vi "RampVoltagewithDDSv11.vi"() -> ()   [LabVIEW 2016]
uses:
  <vilib>/DAQmx/write.llb/DAQmx Write (Digital 1D Wfm NChan NSamp).vi
  <vilib>/DAQmx/write.llb/DAQmx Write (Analog 2D DBL NChan NSamp).vi
  <vilib>/DAQmx/create/channels.llb/DAQmx Create Channel (AO-Voltage-Basic).vi
  <vilib>/DAQmx/create/channels.llb/DAQmx Create Channel (DO-Digital Output).vi
  <vilib>/DAQmx/configure/timing.llb/DAQmx Timing (Sample Clock).vi
  <vilib>/DAQmx/configure/trigger.llb/DAQmx Start Trigger (Digital Edge).vi
  <vilib>/DAQmx/miscellaneous.llb/DAQmx Fill In Error Info.vi
  <vilib>/Waveform/DWDTOps.llb/DWDT Boolean Array to Digital.vi
  <vilib>/Waveform/DWDTOps.llb/DWDT Uncompress Digital.vi
  <vilib>/Waveform/DTblOps.llb/DTbl Digital to Analog.vi
  <resource>/objmgr/daqmx.rc
panel:
  in  "High/Low":bool
  in  "Reset P0.1":bool
  in  "Constant PO.0?":bool
  in  "DDS Trigger delay (ms)":dbl=0.5 step=0.01
  in  "DDS Trigger (Port 0 Line 1)":tag="Dev2/port0/line1"
  out "Digital Output":cluster{i32, dbl, dbl[][]}(graph)={0, 1e-05, [[0.0, 0.0, 0.0, 0.0, 0.0, 0.0, 0.0, 0.0, 0.0, 0.0, 0.0, 0.0, 0.0, 0.0, 0.0, 0.0, 0.0, 0.0, 0.0, 0.0, 0.0, 0.0, 0.0, 0.0, 0.0, 0.0, 0.0, 0.0, 0.0, 0.0, 0.0, 0.0, 0.0, 0.0, 0.0, 0.0, 0.0, 0.0, 0.0, 0.0, 0.0, 0.0, 0.0, 0.0, 0.0, 0.0, 0.0, 0.0, 0.0, 0.0, 0.0, 0.0, 0.0, 0.0, 0.0, 0.0, 0.0, 0.0, 0.0, 0.0, 0.0, 0.0, 0.0, 0.0, 0.0, 0.0, 0.0, 0.0, 0.0, 0.0, 0.0, 0.0, 0.0, 0.0, 0.0, 0.0, 0.0, 0.0, 0.0, 0.0, 0.0, 0.0, 0.0, 0.0, 0.0, 0.0, 0.0, 0.0, 0.0, 0.0, 0.0, 0.0, 0.0, 0.0, 0.0, 0.0, 0.0, 0.0, 0.0, 0.0, 5.0, 5.0, 5.0, 5.0, 5.0, 5.0, 5.0, 5.0, 5.0, 5.0, 5.0, 5.0, 5.0, 5.0, 5.0, 5.0, 5.0, 5.0, 5.0, 5.0, 5.0, 5.0, 5.0, 5.0, 5.0, 5.0, 5.0, 5.0, 5.0, 5.0, 5.0, 5.0, 5.0, 5.0, 5.0, 5.0, 5.0, 5.0, 5.0, 5.0, 5.0, 5.0, 5.0, 5.0, 5.0, 5.0, 5.0, 5.0, 5.0, 5.0, 5.0, 5.0, 5.0, 5.0, 5.0, 5.0, 5.0, 5.0, 5.0, 5.0, 5.0, 5.0, 5.0, 5.0, 5.0, 5.0, 5.0, 5.0, 5.0, 5.0, 5.0, 5.0, 5.0, 5.0, 5.0, 5.0, 5.0, 5.0, 5.0, 5.0, 5.0, 5.0, 5.0, 5.0, 5.0, 5.0, 5.0, 5.0, 5.0, 5.0, 5.0, 5.0, 5.0, 5.0, 5.0, 5.0, 5.0, 5.0, 5.0, 5.0, 5.0, 5.0, 5.0, 5.0, 5.0, 5.0, 5.0, 5.0, 5.0, 5.0, 5.0, 5.0, 5.0, 5.0, 5.0, 5.0, 5.0, 5.0, 5.0, 5.0, 5.0, 5.0, 5.0, 5.0, 5.0, 5.0, 5.0, 5.0, 5.0, 5.0, 5.0, 5.0, 5.0, 5.0, 5.0, 5.0, 5.0, 5.0, 5.0, 5.0, 5.0, 5.0, 5.0, 5.0, 5.0, 5.0, 5.0, 5.0, 5.0, 5.0, 5.0, 5.0, 5.0, 5.0, 5.0, 5.0, 5.0, 5.0, 5.0, 5.0, 5.0, 5.0, 5.0, 5.0, 5.0, 5.0, 5.0, 5.0, 5.0, 5.0, 5.0, 5.0, 5.0, 5.0, 5.0, 5.0, 5.0, 5.0, 5.0, 5.0, 5.0, 5.0, 5.0, 5.0, 5.0, 5.0, 5.0, 5.0, 5.0, 5.0, 5.0, 5.0, 5.0, 5.0, 5.0, 5.0, 5.0, 5.0, 5.0, 5.0, 0.0, 0.0, 0.0, 0.0, 0.0, 0.0, 0.0, 0.0, 0.0, 0.0, 0.0, 0.0, 0.0, 0.0, 0.0, 0.0, 0.0, 0.0, 0.0, 0.0, 0.0, 0.0, 0.0, 0.0, 0.0, 0.0, 0.0, 0.0, 0.0, 0.0, 0.0, 0.0, 0.0, 0.0, 0.0, 0.0, 0.0, 0.0, 0.0, 0.0, 0.0, 0.0, 0.0, 0.0, 0.0, 0.0, 0.0, 0.0, 0.0, 0.0, 0.0, 0.0, 0.0, 0.0, 0.0, 0.0, 0.0, 0.0, 0.0, 0.0, 0.0, 0.0, 0.0, 0.0, 0.0, 0.0, 0.0, 0.0, 0.0, 0.0, 0.0, 0.0, 0.0, 0.0, 0.0, 0.0, 0.0, 0.0, 0.0, 0.0, 0.0, 0.0, 0.0, 0.0, 0.0, 0.0, 0.0, 0.0, 0.0, 0.0, 0.0, 0.0, 0.0, 0.0, 0.0, 0.0, 0.0, 0.0, 0.0, 0.0, 0.0, 0.0, 0.0, 0.0, 0.0, 0.0, 0.0, 0.0, 0.0, 0.0, 0.0, 0.0, 0.0, 0.0, 0.0, 0.0, 0.0, 0.0, 0.0, 0.0, 0.0, 0.0, 0.0, 0.0, 0.0, 0.0, 0.0, 0.0, 0.0, 0.0, 0.0, 0.0, 0.0, 0.0, 0.0, 0.0, 0.0, 0.0, 0.0, 0.0, 0.0, 0.0, 0.0, 0.0, 0.0, 0.0, 0.0, 0.0, 0.0, 0.0, 0.0, 0.0, 0.0, 0.0, 0.0, 0.0, 0.0, 0.0, 0.0, 0.0, 0.0, 0.0, 0.0, 0.0, 0.0, 0.0, 0.0, 0.0, 0.0, 0.0, 0.0, 0.0, 0.0, 0.0, 0.0, 0.0, 0.0, 0.0, 0.0, 0.0, 0.0, 0.0, 0.0, 0.0, 0.0, 0.0, 0.0, 0.0, 0.0, 0.0, 0.0, 0.0, 0.0, 0.0, 0.0, 0.0, 0.0, 0.0, 0.0, 0.0, 5.0, 5.0, 5.0, 5.0, 5.0, 5.0, 5.0, 5.0, 5.0, 5.0, 5.0, 5.0, 5.0, 5.0, 5.0, 5.0, 5.0, 5.0, 5.0, 5.0, 5.0, 5.0, 5.0, 5.0, 5.0, 5.0, 5.0, 5.0, 5.0, 5.0, 5.0, 5.0, 5.0, 5.0, 5.0, 5.0, 5.0, 5.0, 5.0, 5.0, 5.0, 5.0, 5.0, 5.0, 5.0, 5.0, 5.0, 5.0, 5.0, 5.0, 5.0, 5.0, 5.0, 5.0, 5.0, 5.0, 5.0, 5.0, 5.0, 5.0, 5.0, 5.0, 5.0, 5.0, 5.0, 5.0, 5.0, 5.0, 5.0, 5.0, 5.0, 5.0, 5.0, 5.0, 5.0, 5.0, 5.0, 5.0, 5.0, 5.0, 5.0, 5.0, 5.0, 5.0, 5.0, 5.0, 5.0, 5.0, 5.0, 5.0, 5.0, 5.0, 5.0, 5.0, 5.0, 5.0, 5.0, 5.0, 5.0, 5.0, 5.0, 5.0, 5.0, 5.0, 5.0, 5.0, 5.0, 5.0, 5.0, 5.0, 5.0, 5.0, 5.0, 5.0, 5.0, 5.0, 5.0, 5.0, 5.0, 5.0, 5.0, 5.0, 5.0, 5.0, 5.0, 5.0, 5.0, 5.0, 5.0, 5.0, 5.0, 5.0, 5.0, 5.0, 5.0, 5.0, 5.0, 5.0, 5.0, 5.0, 5.0, 5.0, 5.0, 5.0, 5.0, 5.0, 5.0, 5.0, 5.0, 5.0, 5.0, 5.0, 5.0, 5.0, 5.0, 5.0, 5.0, 5.0, 5.0, 5.0, 5.0, 5.0, 5.0, 5.0, 5.0, 5.0, 5.0, 5.0, 5.0, 5.0, 5.0, 5.0, 5.0, 5.0, 5.0, 5.0, 5.0, 5.0, 5.0, 5.0, 5.0, 5.0, 5.0, 5.0, 5.0, 5.0, 5.0, 5.0, 5.0, 5.0, 5.0, 5.0, 5.0, 5.0, 5.0, 5.0, 5.0, 5.0, 5.0, 5.0, 0.0, 0.0, 0.0, 0.0, 0.0, 0.0, 0.0, 0.0, 0.0, 0.0, 0.0, 0.0, 0.0, 0.0, 0.0, 0.0, 0.0, 0.0, 0.0, 0.0, 0.0, 0.0, 0.0, 0.0, 0.0, 0.0, 0.0, 0.0, 0.0, 0.0, 0.0, 0.0, 0.0, 0.0, 0.0, 0.0, 0.0, 0.0, 0.0, 0.0, 0.0, 0.0, 0.0, 0.0, 0.0, 0.0, 0.0, 0.0, 0.0, 0.0, 0.0, 0.0, 0.0, 0.0, 0.0, 0.0, 0.0, 0.0, 0.0, 0.0, 0.0, 0.0, 0.0, 0.0, 0.0, 0.0, 0.0, 0.0, 0.0, 0.0, 0.0, 0.0, 0.0, 0.0, 0.0, 0.0, 0.0, 0.0, 0.0, 0.0, 0.0, 0.0, 0.0, 0.0, 0.0, 0.0, 0.0, 0.0, 0.0, 0.0, 0.0, 0.0, 0.0, 0.0, 0.0, 0.0, 0.0, 0.0, 0.0, 0.0, 5.0], [5.0, 5.0, 5.0, 5.0, 5.0, 5.0, 5.0, 5.0, 5.0, 5.0, 5.0, 5.0, 5.0, 5.0, 5.0, 5.0, 5.0, 5.0, 5.0, 5.0, 5.0, 5.0, 5.0, 5.0, 5.0, 5.0, 5.0, 5.0, 5.0, 5.0, 5.0, 5.0, 5.0, 5.0, 5.0, 5.0, 5.0, 5.0, 5.0, 5.0, 5.0, 5.0, 5.0, 5.0, 5.0, 5.0, 5.0, 5.0, 5.0, 5.0, 5.0, 5.0, 5.0, 5.0, 5.0, 5.0, 5.0, 5.0, 5.0, 5.0, 5.0, 5.0, 5.0, 5.0, 5.0, 5.0, 5.0, 5.0, 5.0, 5.0, 5.0, 5.0, 5.0, 5.0, 5.0, 5.0, 5.0, 5.0, 5.0, 5.0, 5.0, 5.0, 5.0, 5.0, 5.0, 5.0, 5.0, 5.0, 5.0, 5.0, 5.0, 5.0, 5.0, 5.0, 5.0, 5.0, 5.0, 5.0, 5.0, 5.0, 5.0, 5.0, 5.0, 5.0, 5.0, 5.0, 5.0, 5.0, 5.0, 5.0, 5.0, 5.0, 5.0, 5.0, 5.0, 5.0, 5.0, 5.0, 5.0, 5.0, 5.0, 5.0, 5.0, 5.0, 5.0, 5.0, 5.0, 5.0, 5.0, 5.0, 5.0, 5.0, 5.0, 5.0, 5.0, 5.0, 5.0, 5.0, 5.0, 5.0, 5.0, 5.0, 5.0, 5.0, 5.0, 5.0, 5.0, 5.0, 5.0, 5.0, 0.0, 0.0, 0.0, 0.0, 0.0, 0.0, 0.0, 0.0, 0.0, 0.0, 0.0, 0.0, 0.0, 0.0, 0.0, 0.0, 0.0, 0.0, 0.0, 0.0, 0.0, 0.0, 0.0, 0.0, 0.0, 0.0, 0.0, 0.0, 0.0, 0.0, 0.0, 0.0, 0.0, 0.0, 0.0, 0.0, 0.0, 0.0, 0.0, 0.0, 0.0, 0.0, 0.0, 0.0, 0.0, 0.0, 0.0, 0.0, 0.0, 0.0, 0.0, 0.0, 0.0, 0.0, 0.0, 0.0, 0.0, 0.0, 0.0, 0.0, 0.0, 0.0, 0.0, 0.0, 0.0, 0.0, 0.0, 0.0, 0.0, 0.0, 0.0, 0.0, 0.0, 0.0, 0.0, 0.0, 0.0, 0.0, 0.0, 0.0, 0.0, 0.0, 0.0, 0.0, 0.0, 0.0, 0.0, 0.0, 0.0, 0.0, 0.0, 0.0, 0.0, 0.0, 0.0, 0.0, 0.0, 0.0, 0.0, 0.0, 0.0, 0.0, 0.0, 0.0, 0.0, 0.0, 0.0, 0.0, 0.0, 0.0, 0.0, 0.0, 0.0, 0.0, 0.0, 0.0, 0.0, 0.0, 0.0, 0.0, 0.0, 0.0, 0.0, 0.0, 0.0, 0.0, 0.0, 0.0, 0.0, 0.0, 0.0, 0.0, 0.0, 0.0, 0.0, 0.0, 0.0, 0.0, 0.0, 0.0, 0.0, 0.0, 0.0, 0.0, 0.0, 0.0, 0.0, 0.0, 0.0, 0.0, 0.0, 0.0, 0.0, 0.0, 0.0, 0.0, 0.0, 0.0, 0.0, 0.0, 0.0, 0.0, 0.0, 0.0, 0.0, 0.0, 0.0, 0.0, 0.0, 0.0, 0.0, 0.0, 0.0, 0.0, 0.0, 0.0, 0.0, 0.0, 0.0, 0.0, 0.0, 0.0, 0.0, 0.0, 0.0, 0.0, 0.0, 0.0, 0.0, 0.0, 0.0, 0.0, 0.0, 0.0, 0.0, 0.0, 0.0, 0.0, 0.0, 0.0, 0.0, 0.0, 0.0, 0.0, 0.0, 0.0, 0.0, 0.0, 0.0, 0.0, 0.0, 0.0, 0.0, 0.0, 0.0, 0.0, 0.0, 0.0, 0.0, 0.0, 0.0, 0.0, 0.0, 0.0, 0.0, 0.0, 0.0, 0.0, 0.0, 0.0, 0.0, 0.0, 0.0, 0.0, 0.0, 0.0, 0.0, 0.0, 0.0, 0.0, 0.0, 0.0, 0.0, 0.0, 0.0, 0.0, 0.0, 0.0, 0.0, 0.0, 0.0, 0.0, 0.0, 0.0, 0.0, 0.0, 0.0, 0.0, 0.0, 0.0, 0.0, 0.0, 0.0, 0.0, 0.0, 0.0, 0.0, 0.0, 0.0, 0.0, 0.0, 0.0, 0.0, 0.0, 0.0, 0.0, 0.0, 0.0, 0.0, 0.0, 0.0, 0.0, 0.0, 0.0, 0.0, 0.0, 0.0, 0.0, 0.0, 0.0, 0.0, 0.0, 0.0, 0.0, 0.0, 0.0, 0.0, 0.0, 0.0, 0.0, 0.0, 0.0, 0.0, 0.0, 0.0, 0.0, 0.0, 0.0, 0.0, 0.0, 0.0, 0.0, 0.0, 0.0, 0.0, 0.0, 0.0, 0.0, 0.0, 0.0, 0.0, 0.0, 0.0, 0.0, 0.0, 0.0, 0.0, 0.0, 0.0, 0.0, 0.0, 0.0, 0.0, 0.0, 0.0, 0.0, 0.0, 0.0, 0.0, 0.0, 0.0, 0.0, 0.0, 0.0, 0.0, 0.0, 0.0, 0.0, 0.0, 0.0, 0.0, 0.0, 0.0, 0.0, 0.0, 0.0, 0.0, 0.0, 0.0, 0.0, 0.0, 0.0, 0.0, 0.0, 0.0, 0.0, 0.0, 0.0, 0.0, 0.0, 0.0, 0.0, 0.0, 0.0, 0.0, 0.0, 0.0, 0.0, 0.0, 0.0, 0.0, 0.0, 0.0, 0.0, 0.0, 0.0, 0.0, 0.0, 0.0, 0.0, 0.0, 0.0, 0.0, 0.0, 0.0, 0.0, 0.0, 0.0, 0.0, 0.0, 0.0, 0.0, 0.0, 0.0, 0.0, 0.0, 0.0, 0.0, 0.0, 0.0, 0.0, 0.0, 0.0, 0.0, 0.0, 0.0, 0.0, 0.0, 0.0, 0.0, 0.0, 0.0, 0.0, 0.0, 0.0, 0.0, 0.0, 0.0, 0.0, 0.0, 0.0, 0.0, 0.0, 0.0, 0.0, 0.0, 0.0, 0.0, 0.0, 0.0, 0.0, 0.0, 0.0, 0.0, 0.0, 0.0, 0.0, 0.0, 0.0, 0.0, 0.0, 0.0, 0.0, 0.0, 0.0, 0.0, 0.0, 0.0, 0.0, 0.0, 0.0, 0.0, 0.0, 0.0, 0.0, 0.0, 0.0, 0.0, 0.0, 0.0, 0.0, 0.0, 0.0, 0.0, 0.0, 0.0, 0.0, 0.0, 0.0, 0.0, 0.0, 0.0, 0.0, 0.0, 0.0, 0.0, 0.0, 0.0, 0.0, 0.0, 0.0, 0.0, 0.0, 0.0, 0.0, 0.0, 0.0, 0.0, 0.0, 0.0, 0.0, 0.0, 0.0, 0.0, 0.0, 0.0, 0.0, 0.0, 0.0, 0.0, 0.0, 0.0, 0.0, 0.0, 0.0, 0.0, 0.0, 0.0, 0.0, 0.0, 0.0, 0.0, 0.0, 0.0, 0.0, 0.0, 0.0, 0.0, 0.0, 0.0, 0.0, 0.0, 0.0, 0.0, 0.0, 0.0, 0.0, 0.0, 0.0, 0.0, 0.0, 0.0, 0.0, 0.0, 0.0, 0.0, 0.0, 0.0, 0.0, 0.0, 0.0, 0.0, 0.0, 0.0, 0.0, 0.0, 0.0, 0.0, 0.0, 0.0, 0.0, 0.0, 0.0, 0.0, 0.0, 0.0, 0.0, 0.0, 0.0, 0.0, 0.0, 0.0, 0.0, 0.0, 0.0, 0.0, 0.0, 0.0, 0.0, 0.0, 0.0, 0.0, 0.0, 0.0, 0.0, 0.0, 0.0, 0.0, 0.0, 0.0, 0.0, 0.0, 0.0, 0.0, 0.0, 0.0, 0.0, 0.0, 0.0, 0.0, 0.0, 0.0, 0.0, 0.0, 0.0, 0.0, 0.0, 0.0, 0.0, 0.0, 0.0, 0.0, 0.0, 0.0, 0.0, 0.0, 0.0, 0.0, 0.0, 0.0, 0.0, 0.0, 0.0, 0.0, 0.0, 0.0, 0.0, 0.0, 0.0, 0.0, 0.0, 0.0, 0.0, 0.0, 0.0, 0.0, 0.0, 0.0, 0.0, 0.0, 0.0, 0.0, 0.0, 0.0, 0.0, 0.0, 0.0, 0.0, 0.0, 0.0, 5.0]]}
  out "Analog Outputs":cluster{i32, dbl, dbl[][]}(graph)={0, 4e-06, array4x2001[8004 elements]}
  in  "Phase Lock Switch (Port 0 Line 0)":tag="Dev2/port0/line0"
  in  "Ramp to phase lock\n switch delay (ms)":dbl step=0.01
  in  "error in 2":errorcluster caption="error in"
  in  "ao3 ramp amplitude (V)":dbl
  in  "ao2 ramp amplitude (V)":dbl
  in  "ao1 ramp amplitude (V)":dbl
  in  "SolsTiS 2 - Fast Piezo (ao3)":tag="Dev2/ao3"
  in  "SolsTiS 2 - Slow Piezo (ao2)":tag="Dev2/ao2"
  out "size(s)":i32=2001
  in  "Trigger delay NI (ms)":dbl=1.0
  in  "Trigger Input (PFI0)":tag="/Dev2/PFI0"
  in  "SolsTiS 1 - Fast Piezo (ao1)":tag="Dev2/ao1"
  in  "SolsTiS 1 - Slow Piezo (ao0)":tag="Dev2/ao0"
  in  "Plateau duration (ms)":dbl=2.0 step=0.01
  in  "Ramp duration (ms)":dbl=2.0 step=0.01
  in  "ao0 ramp amplitude (V)":dbl=0.09 step=0.001
  in  "error in":errorcluster
  # "MAGIS LASER SYSTEM\nChirp Control"
  # "Ramp Definition"
  # "Output Monitor"
  # "Channel Definition"
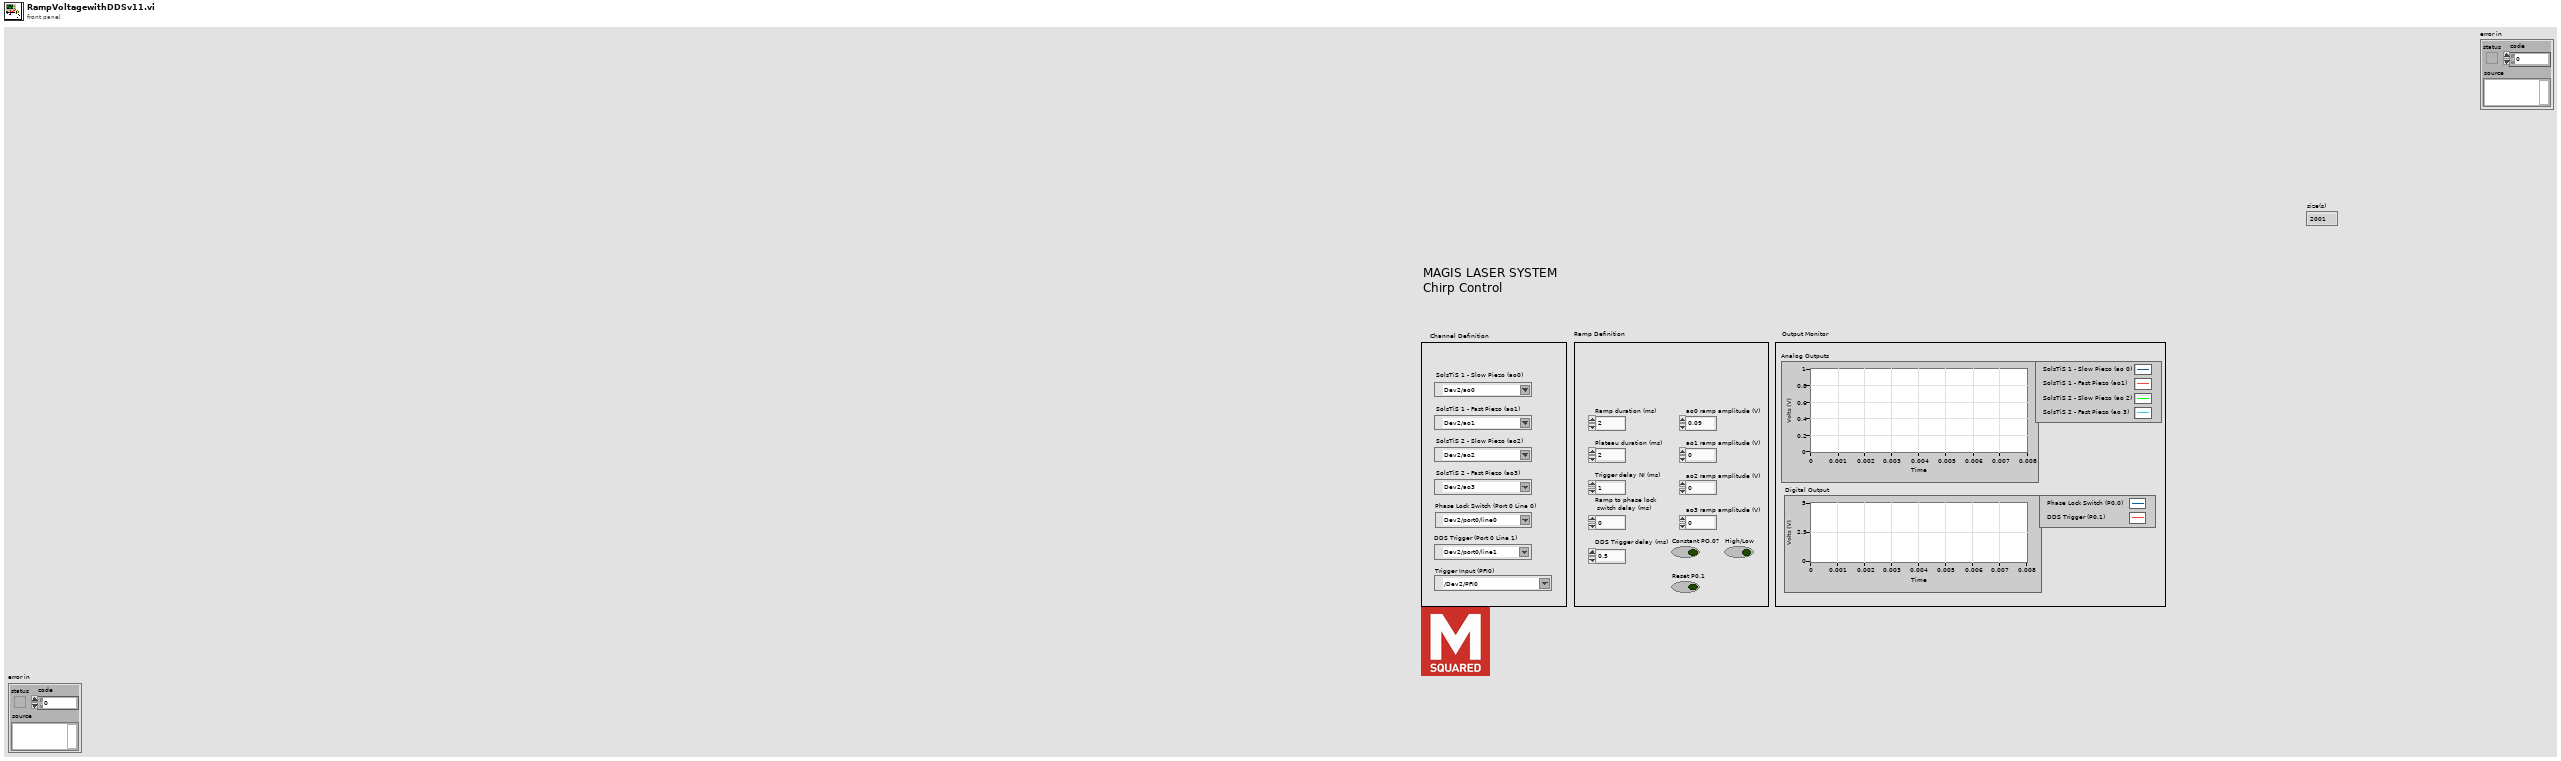
[diagram p1: front panel]
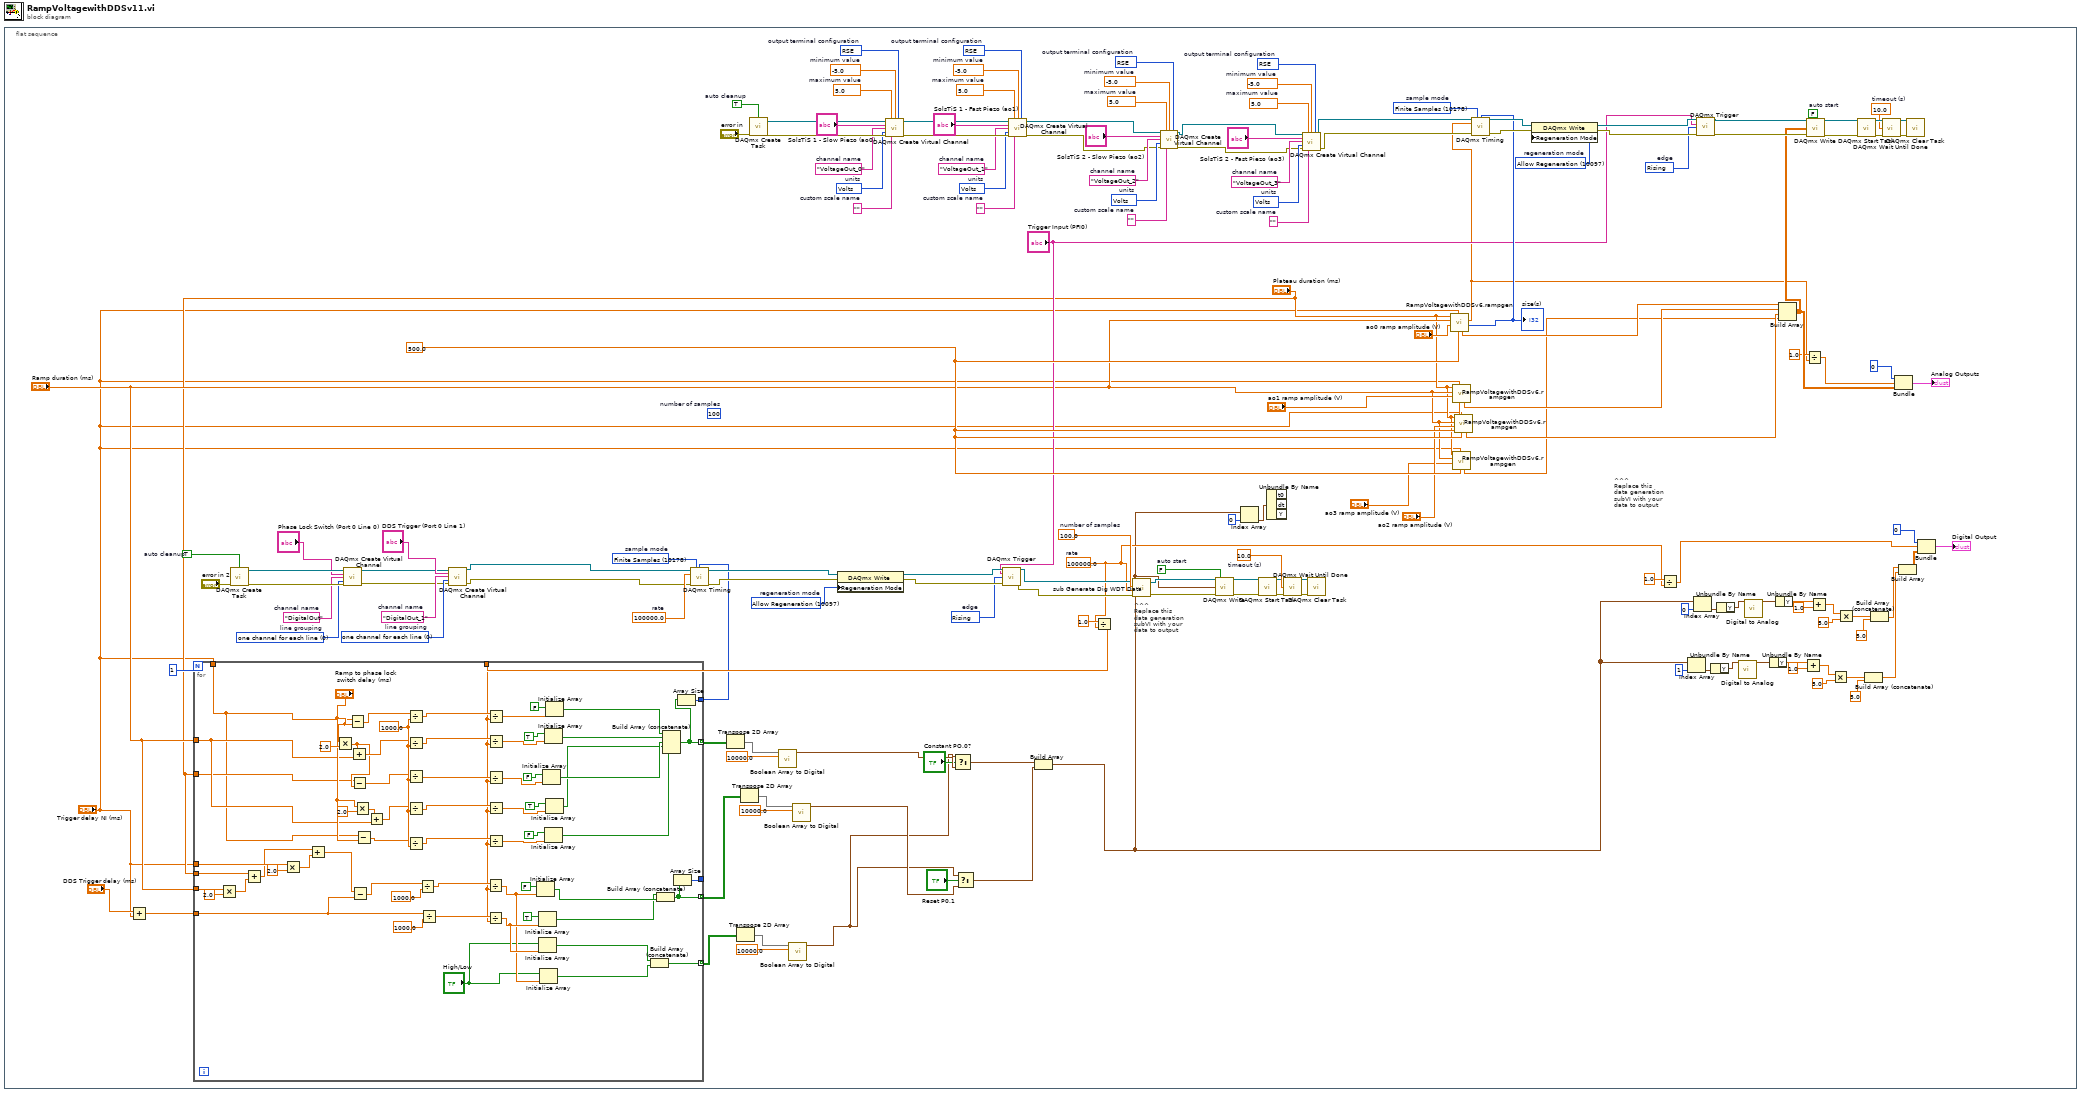
[diagram p0: block diagram]
diagram:
  n1 = flat-sequence {
    frame #0 {
      w37 = 0 items=["one channel for each line", "one channel for all lines"]  # line grouping
      w36 = "DigitalOut_1"  # channel name
      w105 = 500.0 ("No of samples in ramp (500 or less)")
      w72 = 10280 items=["Rising"=10280, "Falling"=10171]  # edge
      w74 = 10097 items=["Allow Regeneration"=10097, "Do Not Allow Regeneration"=10158]  # regeneration mode
      w77 = 10178 items=["Finite Samples"=10178, "Continuous Samples"=10123, "Hardware Timed Single Point"=12522]  # sample mode
      (unwired) 100  # number of samples
      w78 = 100000.0  # rate
      w81 = 0 items=["one channel for each line", "one channel for all lines"]  # line grouping
      w80 = "DigitalOut"  # channel name
      w83 = TRUE  # auto cleanup
      w98 = 10.0  # timeout (s)
      w46 = 100000.0  # rate
      w91 = 100.0  # number of samples
      w88 = FALSE  # auto start
      w112 = 10083 items=["Default"=-1, "RSE"=10083, "Differential"=10106, "Pseudodifferential"=12529]  # output terminal configuration
      w113 = 10348 items=["Volts"=10348, "From Custom Scale"=10065]  # units
      w114 = "VoltageOut_3"  # channel name
      w115 = ""  # custom scale name
      w116 = -5.0  # minimum value
      w117 = 5.0  # maximum value
      w121 = 10083 items=["Default"=-1, "RSE"=10083, "Differential"=10106, "Pseudodifferential"=12529]  # output terminal configuration
      w122 = 10348 items=["Volts"=10348, "From Custom Scale"=10065]  # units
      w123 = "VoltageOut_2"  # channel name
      w124 = ""  # custom scale name
      w125 = -5.0  # minimum value
      w126 = 5.0  # maximum value
      w133 = 10280 items=["Rising"=10280, "Falling"=10171]  # edge
      w135 = 10097 items=["Allow Regeneration"=10097, "Do Not Allow Regeneration"=10158]  # regeneration mode
      w138 = 10178 items=["Finite Samples"=10178, "Continuous Samples"=10123, "Hardware Timed Single Point"=12522]  # sample mode
      w140 = 10083 items=["Default"=-1, "RSE"=10083, "Differential"=10106, "Pseudodifferential"=12529]  # output terminal configuration
      w141 = 10348 items=["Volts"=10348, "From Custom Scale"=10065]  # units
      w142 = "VoltageOut_1"  # channel name
      w143 = ""  # custom scale name
      w144 = -5.0  # minimum value
      w145 = 5.0  # maximum value
      w147 = 10083 items=["Default"=-1, "RSE"=10083, "Differential"=10106, "Pseudodifferential"=12529]  # output terminal configuration
      w148 = 10348 items=["Volts"=10348, "From Custom Scale"=10065]  # units
      w149 = "VoltageOut_0"  # channel name
      w151 = ""  # custom scale name
      w152 = -5.0  # minimum value
      w153 = 5.0  # maximum value
      w155 = TRUE  # auto cleanup
      w161 = 10.0  # timeout (s)
      w165 = FALSE  # auto start
      # "^^^\nReplace this\ndata generation\nsubVI with your\ndata to output"
      # "^^^\nReplace this\ndata generation\nsubVI with your\ndata to output"
      n2 = Add(x="DDS Trigger delay (ms)", y="Trigger delay NI (ms)") -> (x+y=w31:dbl)
      n3 = call <vilib>:"DAQmx Create Task.vi"("auto cleanup"=w83, "error in"="error in 2") -> ("task out"=w82:refnum<k21>, "error out"=w84:errorcluster)  [unwired: 12 in]
      n4 = call-poly <vilib>:"DAQmx Create Virtual Channel.vi"("task in"=w82, "lines"="Phase Lock Switch (Port 0 Line 0)", "name to assign"=w80, "line grouping"=w81, "error in"=w84) -> ("task out"=w33:refnum<k21>, "error out"=w34:errorcluster)  [unwired: 9 in]
      n5 = call-poly <vilib>:"DAQmx Create Virtual Channel.vi"("task in"=w33, "lines"="DDS Trigger (Port 0 Line 1)", "name to assign"=w36, "line grouping"=w37, "error in"=w34) -> ("task out"=w2:refnum<k21>, "error out"=w1:errorcluster)  [unwired: 9 in]
      n6 = call <vilib>:"DAQmx Create Task.vi"("auto cleanup"=w155, "error in"="error in") -> ("task out"=w154:refnum<k21>, "error out"=w156:errorcluster)  [unwired: 12 in]
      n7 = call-poly <vilib>:"DAQmx Create Virtual Channel.vi"("task in"=w154, "maximum value"=w153, "minimum value"=w152, "output terminal configuration"=w147, "physical channels"="SolsTiS 1 - Slow Piezo (ao0)", "name to assign"=w149, "units"=w148, "error in"=w156, "custom scale name"=w151) -> ("task out"=w146:refnum<k21>, "error out"=w150:errorcluster)  [unwired: 5 in]
      n8 = call-poly <vilib>:"DAQmx Create Virtual Channel.vi"("task in"=w146, "maximum value"=w145, "minimum value"=w144, "output terminal configuration"=w140, "physical channels"="SolsTiS 1 - Fast Piezo (ao1)", "name to assign"=w142, "units"=w141, "error in"=w150, "custom scale name"=w143) -> ("task out"=w119:refnum<k21>, "error out"=w118:errorcluster)  [unwired: 5 in]
      n9 = Divide(x=1.0, y=w46) -> (x/y=w68:dbl)
      n10 = for {
        N: 1 -> [_]
        tunnel: w68 -> [w181]
        tunnel: [w208] -> w65 mode=indexing
        tunnel: [w207] -> w64
        tunnel: "Ramp duration (ms)" -> [w196]
        tunnel: "Plateau duration (ms)" -> [w195]
        tunnel: "Trigger delay NI (ms)" -> [w194]
        tunnel: w31 -> [w187]
        tunnel: "Ramp duration (ms)" -> [w191]
        tunnel: "Plateau duration (ms)" -> [w188]
        tunnel: [w178] -> _
        tunnel: "Trigger delay NI (ms)" -> [w175]
        tunnel: [w172] -> w25 mode=indexing
        tunnel: [w168] -> w22 mode=indexing
        w227 = 1000.0
        n11 = Multiply(x=w191, y=2.0) -> (x*y=w189:dbl)
        n12 = Add(x=w188, y=w189) -> (x+y=w174:dbl)
        n13 = Multiply(x=w175, y=2.0) -> (x*y=w176:dbl)
        n14 = Add(x=w174, y=w176) -> (x+y=w173:dbl)
        n15 = Multiply(x="Ramp to phase lock\n switch delay (ms)", y=2.0) -> (x*y=w203:dbl)
        n16 = Subtract(x=w194, y="Ramp to phase lock\n switch delay (ms)") -> (x-y=w206:dbl)
        n17 = Add(x=w203, y=w196) -> (x+y=w204:dbl)
        n18 = Subtract(x=w195, y=w203) -> (x-y=w202:dbl)
        n19 = Subtract(x=w173, y=w187) -> (x-y=w184:dbl)
        n20 = Multiply(x="Ramp to phase lock\n switch delay (ms)", y=2.0) -> (x*y=w200:dbl)
        n21 = Subtract(x=w194, y="Ramp to phase lock\n switch delay (ms)") -> (x-y=w197:dbl)
        n22 = Add(x=w200, y=w196) -> (x+y=w199:dbl)
        n23 = Divide(x=w206, y=w227) -> (x/y=w226:dbl)
        n24 = Divide(x=w204, y=w227) -> (x/y=w225:dbl)
        n25 = Divide(x=w202, y=w227) -> (x/y=w224:dbl)
        n26 = Divide(x=w199, y=w227) -> (x/y=w223:dbl)
        n27 = Divide(x=w197, y=w227) -> (x/y=w222:dbl)
        n28 = Divide(x=w184, y=1000.0) -> (x/y=w183:dbl)
        n29 = Divide(x=w187, y=1000.0) -> (x/y=w182:dbl)
        n30 = Divide(x=w183, y=w181) -> (x/y=w167:dbl)
        n31 = Divide(x=w182, y=w181) -> (x/y=w171:dbl)
        n32 = Divide(x=w226, y=w181) -> (x/y=w218:dbl)
        n33 = Divide(x=w225, y=w181) -> (x/y=w217:dbl)
        n34 = Divide(x=w224, y=w181) -> (x/y=w216:dbl)
        n35 = Divide(x=w223, y=w181) -> (x/y=w215:dbl)
        n36 = Divide(x=w222, y=w181) -> (x/y=w214:dbl)
        n37 = Initialize Array(FALSE, w167) -> (w180:bool[])
        n38 = Initialize Array(TRUE, w171) -> (w179:bool[])
        n39 = Initialize Array("High/Low", w171) -> (w170:bool[])
        n40 = Initialize Array("High/Low", w167) -> (w169:bool[])
        n41 = Initialize Array(FALSE, w216) -> (w211:bool[])
        n42 = Initialize Array(TRUE, w217) -> (w212:bool[])
        n43 = Initialize Array(FALSE, w214) -> (w209:bool[])
        n44 = Initialize Array(FALSE, w218) -> (w213:bool[])
        n45 = Initialize Array(TRUE, w215) -> (w210:bool[])
        n46 = Build Array (concatenate)(w170, w169) -> (w168:bool[])
        n47 = Build Array (concatenate)(w179, w180) -> (w172:bool[])
        n48 = Build Array (concatenate)(w213, w212, w211, w210, w209) -> (w208:bool[])
        n49 = Array Size(array=w172) -> (size(s)=w178:i32)
        n50 = Array Size(array=w208) -> (size(s)=w207:i32)
      }
      n51 = call-poly <vilib>:"DAQmx Timing.vi"("task/channels in"=w2, "sample mode"=w77, "samples per channel"=w64, "rate"=w78, "error in"=w1) -> ("task out"=w76:refnum<k21>, "error out"=w79:errorcluster)  [unwired: 9 in]
      n52 = Transpose 2D Array(2D array=w65) -> (transposed array=w66:bool[][])
      n53 = Transpose 2D Array(2D array=w22) -> (transposed array=w23:bool[][])
      n54 = Transpose 2D Array(2D array=w25) -> (transposed array=w26:bool[][])
      n55 = call-poly <vilib>:"Boolean Array to Digital.vi"("sample rate"=10000.0, "boolean array"=w66) -> ("digital waveform"=w10:digitalwaveform)  [unwired: 8 in, 1 out]
      n56 = call-poly <vilib>:"Boolean Array to Digital.vi"("sample rate"=10000.0, "boolean array"=w23) -> ("digital waveform"=w3:digitalwaveform)  [unwired: 8 in, 1 out]
      n57 = call-poly <vilib>:"Boolean Array to Digital.vi"("sample rate"=10000.0, "boolean array"=w26) -> ("digital waveform"=w7:digitalwaveform)  [unwired: 8 in, 1 out]
      n58 = property class="DAQmx Write"(reference=w76, error in=w79, "Regeneration Mode"=w74) -> (reference out=w73:refnum<k21>, error out=w75:errorcluster)
      n59 = Select(t=w3, s="Constant PO.0?", f=w10) -> (s? t:f=w6:digitalwaveform)
      n60 = Select(t=w3, s="Reset P0.1", f=w7) -> (s? t:f=w5:digitalwaveform)
      n61 = call-poly <vilib>:"DAQmx Trigger.vi"("task/channels in"=w73, "source"="Trigger Input (PFI0)", "edge"=w72, "error in"=w75) -> ("task out"=w71:refnum<k21>, "error out"=w70:errorcluster)  [unwired: 10 in]
      n62 = Build Array(w6, w5) -> (w4:digitalwaveform[])
      n63 = call <vilib>:"sub Generate Dig WDT Data.vi"("task in"=w71, "number of samples"=w91, "update rate"=w46, "error in"=w70) -> ("task out"=w90:refnum<k21>, "error out"=w89:errorcluster)  [unwired: 1 in, 1 out]
      n64 = call-poly <vilib>:"DAQmx Create Virtual Channel.vi"("task in"=w119, "maximum value"=w126, "minimum value"=w125, "output terminal configuration"=w121, "physical channels"="SolsTiS 2 - Slow Piezo (ao2)", "name to assign"=w123, "units"=w122, "error in"=w118, "custom scale name"=w124) -> ("task out"=w110:refnum<k21>, "error out"=w109:errorcluster)  [unwired: 5 in]
      n65 = call-poly <vilib>:"DAQmx Write.vi"("task/channels in"=w90, "auto start"=w88, "data"=w4, "error in"=w89) -> ("task out"=w95:refnum<k21>, "error out"=w96:errorcluster)  [unwired: 9 in, 1 out]
      n66 = Index Array(array=w4, index=0) -> (element=w86:digitalwaveform)
      n67 = call <vilib>:"DAQmx Start Task.vi"("task/channels in"=w95, "error in"=w96) -> ("task out"=w92:refnum<k21>, "error out"=w93:errorcluster)  [unwired: 12 in]
      n68 = Unbundle By Name(w86) -> ()  [unwired: 3 out]
      n69 = call <vilib>:"DAQmx Wait Until Done.vi"("task/channels in"=w92, "timeout (sec)"=w98, "error in"=w93) -> ("task out"=w97:refnum<k21>, "error out"=w94:errorcluster)  [unwired: 11 in]
      n70 = call-poly <vilib>:"DAQmx Create Virtual Channel.vi"("task in"=w110, "maximum value"=w117, "minimum value"=w116, "output terminal configuration"=w112, "physical channels"="SolsTiS 2 - Fast Piezo (ao3)", "name to assign"=w114, "units"=w113, "error in"=w109, "custom scale name"=w115) -> ("task out"=w107:refnum<k21>, "error out"=w108:errorcluster)  [unwired: 5 in]
      n71 = call <vilib>:"DAQmx Clear Task.vi"("task in"=w97, "error in"=w94) -> ()  [unwired: 13 in, 1 out]
      n72 = call "RampVoltagewithDDSv6,rampgen.vi"("No of samples in ramp"=w105, "Trigger delay NI (ms)"="Trigger delay NI (ms)", "Ramp Amplitude (V)}"="ao0 ramp amplitude (V)", "Ramp duration (ms)"="Ramp duration (ms)", "Plateau duration (ms)"="Plateau duration (ms)") -> ("Numeric 2"=w129:i32, "Numeric"=w49:dbl, "Array"=w106:dbl[])  [unwired: 3 in, 1 out]
      "size(s)" <- w129
      n73 = call "RampVoltagewithDDSv6,rampgen.vi"("No of samples in ramp"=w105, "Trigger delay NI (ms)"="Trigger delay NI (ms)", "Ramp Amplitude (V)}"="ao1 ramp amplitude (V)", "Ramp duration (ms)"="Ramp duration (ms)", "Plateau duration (ms)"="Plateau duration (ms)") -> ("Array"=w101:dbl[])  [unwired: 3 in, 3 out]
      n74 = call "RampVoltagewithDDSv6,rampgen.vi"("No of samples in ramp"=w105, "Trigger delay NI (ms)"="Trigger delay NI (ms)", "Ramp Amplitude (V)}"="ao3 ramp amplitude (V)", "Ramp duration (ms)"="Ramp duration (ms)", "Plateau duration (ms)"="Plateau duration (ms)") -> ("Array"=w99:dbl[])  [unwired: 3 in, 3 out]
      n75 = call "RampVoltagewithDDSv6,rampgen.vi"("No of samples in ramp"=w105, "Trigger delay NI (ms)"="Trigger delay NI (ms)", "Ramp Amplitude (V)}"="ao2 ramp amplitude (V)", "Ramp duration (ms)"="Ramp duration (ms)", "Plateau duration (ms)"="Plateau duration (ms)") -> ("Array"=w100:dbl[])  [unwired: 3 in, 3 out]
      n76 = call-poly <vilib>:"DAQmx Timing.vi"("task/channels in"=w107, "sample mode"=w138, "samples per channel"=w129, "rate"=w49, "error in"=w108) -> ("task out"=w137:refnum<k21>, "error out"=w139:errorcluster)  [unwired: 9 in]
      n77 = property class="DAQmx Write"(reference=w137, error in=w139, "Regeneration Mode"=w135) -> (reference out=w134:refnum<k21>, error out=w136:errorcluster)
      n78 = Divide(x=1.0, y=w46) -> (x/y=w45:dbl)
      n79 = Index Array(array=w4, index=1) -> (element=w20:digitalwaveform)
      n80 = Index Array(array=w4, index=0) -> (element=w56:digitalwaveform)
      n81 = call-poly <vilib>:"DAQmx Trigger.vi"("task/channels in"=w134, "source"="Trigger Input (PFI0)", "edge"=w133, "error in"=w136) -> ("task out"=w131:refnum<k21>, "error out"=w130:errorcluster)  [unwired: 10 in]
      n82 = Unbundle By Name(w20) -> ("Y"=w19:digitaldata)
      n83 = Unbundle By Name(w56) -> ("Y"=w55:digitaldata)
      n84 = call-poly <vilib>:"Digital to Analog.vi"("digital table"=w19) -> ("analog waveform"=w18:waveform(dbl))  [unwired: 7 in, 3 out]
      n85 = call-poly <vilib>:"Digital to Analog.vi"("digital table"=w55) -> ("analog waveform"=w54:waveform(dbl))  [unwired: 7 in, 3 out]
      n86 = Unbundle By Name(w18) -> ("Y"=w16:dbl[])
      n87 = Unbundle By Name(w54) -> ("Y"=w43:dbl[])
      n88 = Build Array(w106, w101, w100, w99) -> (w60:dbl[][])
      n89 = Add(x=w16, y=1.0) -> (x+y=w15:dbl[])
      n90 = Divide(x=1.0, y=w49) -> (x/y=w48:dbl)
      n91 = call-poly <vilib>:"DAQmx Write.vi"("task/channels in"=w131, "auto start"=w165, "data"=w60, "error in"=w130) -> ("task out"=w160:refnum<k21>, "error out"=w159:errorcluster)  [unwired: 9 in, 1 out]
      n92 = Add(x=w43, y=1.0) -> (x+y=w42:dbl[])
      n93 = Multiply(x=w15, y=5.0) -> (x*y=w13:dbl[])
      n94 = Multiply(x=w42, y=5.0) -> (x*y=w40:dbl[])
      n95 = call <vilib>:"DAQmx Start Task.vi"("task/channels in"=w160, "error in"=w159) -> ("task out"=w164:refnum<k21>, "error out"=w163:errorcluster)  [unwired: 12 in]
      n96 = Build Array (concatenate)(w13, 5.0 ("y")) -> (w11:dbl[])
      n97 = Build Array (concatenate)(w40, 5.0 ("y")) -> (w38:dbl[])
      n98 = call <vilib>:"DAQmx Wait Until Done.vi"("task/channels in"=w164, "timeout (sec)"=w161, "error in"=w163) -> ("task out"=w158:refnum<k21>, "error out"=w162:errorcluster)  [unwired: 11 in]
      n99 = Bundle(0, w48, w60) -> (→"Analog Outputs":cluster{i32, dbl, dbl[][]})  [unwired: 1 in]
      n100 = Build Array(w38, w11) -> (w51:dbl[][])
      n101 = call <vilib>:"DAQmx Clear Task.vi"("task in"=w158, "error in"=w162) -> ()  [unwired: 13 in, 1 out]
      n102 = Bundle(0, w45, w51) -> (→"Digital Output":cluster{i32, dbl, dbl[][]})  [unwired: 1 in]
    }
  }
